vi "GE5565 Enable DMA Interrupt (Cluster) Multi.vi"(4 "error in (no error)":errorcluster, 6 "transfer size (1024 bytes)":u32=1024, 7 "VMIC reference in":T1) -> (0 "error out":errorcluster, 3 "VMIC reference out":T1)   [LabVIEW 2019, in "RefMem DMA Engine.lvlib"]
uses:
  RefMem DMA Engine.lvlib
  <vilib>/Instr/_visa.llb/Select Event Type.ctl
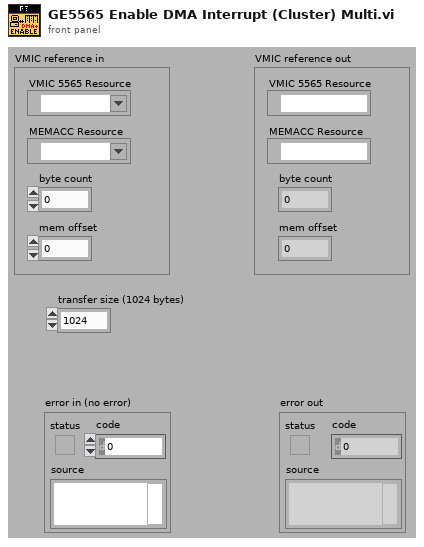
[diagram p1: front panel]
types:
  T1 = cluster{"VMIC 5565 Resource":refnum<visa-resource-name>, "MEMACC Resource":refnum<visa-resource-name>, "byte count":u32, "mem offset":u32}
  T2 = typedef "Select Event Type.ctl" = u32
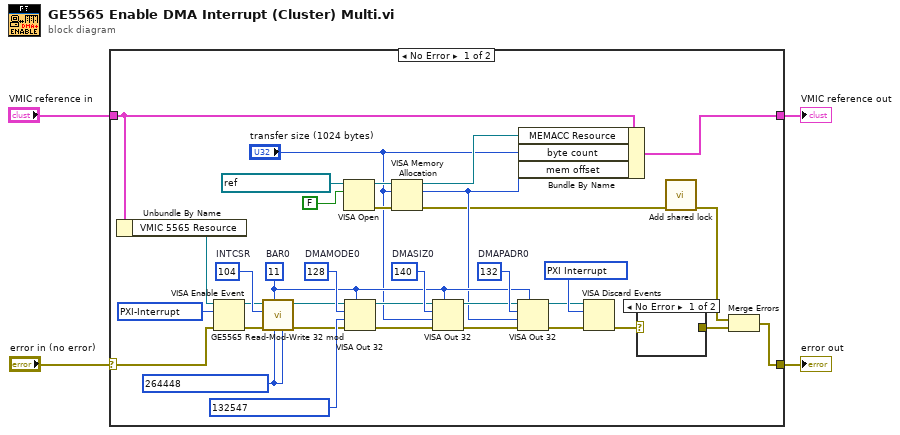
[diagram p0: block diagram]
diagram:
  n1 = case shown="No Error" "error in (no error)" {
    selector: "error in (no error)" -> [w25 w41]
    tunnel: "VMIC reference in" -> [w16 w42]
    tunnel: [w15 w42] -> w1
    tunnel: [w27 w41] -> w3
    frame No Error {
      w23 = u16 11  # BAR0
      w11 = T2 1073684514 items=["Service Request"=1073684491, "Trigger"=3221168138, "Clear"=1073684493, "VXI Signal"=1073684512, "VXI/VME Interrupt"=3221168161, "VXI/VME Sysfail"=1073684509, "VXI/VME Sysreset"=1073684510, "GPIB CIC"=1073684498, "GPIB Talk"=1073684499, "GPIB Listen"=1073684500, "PXI Interrupt"=1073684514, "Serial Break"=1073684515, "Serial TermChar"=1073684516, "Serial CTS"=1073684521, "Serial DSR"=1073684522, "Serial DCD"=1073684524, "Serial RI"=1073684526, "Serial Character"=1073684533, "USB Interrupt"=1073684535, "All Enabled"=1073709055] ("Event Type")
      w24 = u32 104  # INTCSR
      w22 = u32 264448 ("value")
      w26 = T2 1073684514 items=["ServiceRequest"=1073684491, "Trigger"=3221168138, "Clear"=1073684493, "VXI-Signal"=1073684512, "VXI/VME-Interrupt"=3221168161, "VXI/VME-Sysfail"=1073684509, "VXI/VME-Sysreset"=1073684510, "GPIB-CIC"=1073684498, "GPIB-Talk"=1073684499, "GPIB-Listen"=1073684500, "PXI-Interrupt"=1073684514, "AllEnabled"=1073709055] ("Event Type")
      w30 = u32 132  # DMAPADR0
      w33 = u32 140  # DMASIZ0
      w35 = u32 128  # DMAMODE0
      n2 = Unbundle By Name(w16) -> ("VMIC 5565 Resource"=w17:refnum<visa-resource-name>)
      n3 = VISA Enable Event(8:w25, 10:w26, 11:w17) -> (0:w21:errorcluster, 3:w20:refnum<visa-resource-name>)  [unwired: 1 in]
      n4 = call "GE5565 Read-Mod-Write 32 mod.vi"("value"=w22, "inv bit mask"=w22, "address space (13: BAR2)"=w23, "error in (no error)"=w21, "offset (0)"=w24, "VISA resource name"=w20) -> ("error out"=w18:errorcluster, "VISA resource name out"=w19:refnum<visa-resource-name>)  [unwired: 4 in]
      n5 = VISA Open(duplicate session (F)=FALSE, VISA resource name=refnum<visa-resource-name> "PXI0::MEMACC") -> (VISA resource name=w38:refnum<visa-resource-name>, error out=w39:errorcluster)  [unwired: 3 in]
      n6 = VISA Out 32(7:w23, 8:w18, 9:u32 132547 ("value (0)"), 10:w35, 11:w19) -> (0:w32:errorcluster, 3:w31:refnum<visa-resource-name>)
      n7 = VISA Memory Allocation(8:w39, 10:"transfer size (1024 bytes)", 11:w38) -> (0:w6:errorcluster, 2:w14:u32, 3:w13:refnum<visa-resource-name>)
      n8 = VISA Out 32(7:w23, 8:w32, 9:"transfer size (1024 bytes)", 10:w33, 11:w31) -> (0:w28:errorcluster, 3:w29:refnum<visa-resource-name>)
      n9 = VISA Out 32(7:w23, 8:w28, 9:w14, 10:w30, 11:w29) -> (0:w9:errorcluster, 3:w10:refnum<visa-resource-name>)
      n10 = Bundle By Name(cluster=w16, "MEMACC Resource"=w13, "byte count"="transfer size (1024 bytes)", "mem offset"=w14) -> (w15:T1)
      n11 = VISA Discard Events(8:w9, 10:w11, 11:w10) -> (0:w8:errorcluster)  [unwired: 1 in, 1 out]
      n12 = case shown="No Error" w8 {
        selector: w8 -> [_ w40]
        tunnel: [_ w40] -> w7
        frame No Error {
        }
        frame Error {
        }
      }
      n13 = call "Add shared lock.vi"("error in (no error)"=w6) -> ("error out"=w5:errorcluster)  [unwired: 10 in]
      n14 = Merge Errors(w5, w7) -> (w27:errorcluster)
    }
    frame Error {
    }
  }
  "error out" <- w3
  "VMIC reference out" <- w1
